vi "Add Target Library.vi"(8 "error in (no error)":errorcluster, 11 "Builder in":refnum<class "Builder.lvclass">) -> (0 "error out":errorcluster, 3 "Builder out":refnum<class "Builder.lvclass">)   [LabVIEW 2019, in "Builder.lvclass"]
uses:
  Builder.lvclass
  Builder.lvclass/Builder.ctl
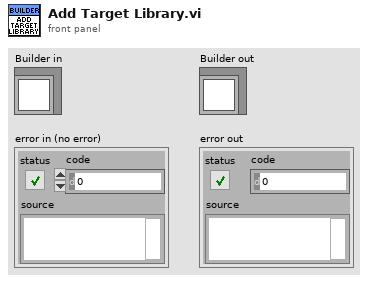
[diagram p1: front panel]
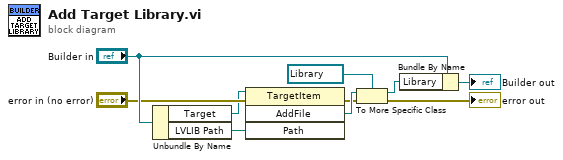
[diagram p0: block diagram]
diagram:
  n1 = Unbundle By Name("Builder in") -> ("Target"=w4:refnum<vi>, "LVLIB Path"=w5:path)
  n2 = invoke class="TargetItem" method="AddFile"(reference=w4, error in="error in (no error)", "Path"=w5) -> (error out=w1:errorcluster, "AddFile"=w2:refnum<vi>)  [unwired: 1 in, 2 out]
  n3 = To More Specific Class(target class=refnum<vi> refnum ("Add File"), reference=w2, error in=w1) -> (specific class reference=w7:refnum<vi>, error out=→"error out":errorcluster)
  n4 = Bundle By Name(cluster="Builder in", "Library"=w7) -> (→"Builder out":refnum<class "Builder.lvclass">)
